vi "solar_write QTimerStopAll.vi"(8 "error in (no error)":errorcluster, 11 "solar in":refnum<class "solar.lvclass">) -> (0 "error out":errorcluster, 2 "Previously Running":bool[](array[boolean]), 3 "solar out":refnum<class "solar.lvclass">)   [LabVIEW 2018, in "solar.lvclass"]
doc: "This stops all QTimers registered and returns if the QTimer was prevously running prior to the stop."
uses:
  solar.lvclass
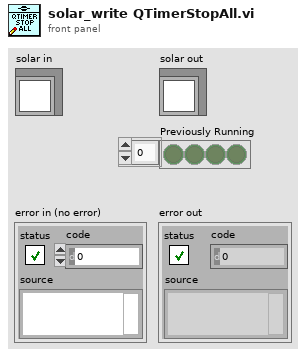
[diagram p1: front panel]
types:
  T1 = typedef "solar_ctl SOLAR Refnum.ctl" = refnum<k1>
  T2 = typedef "solar_ctl SOLAR Global.ctl" = cluster{"Targets":T3[], "AppDir":path, "solar.ini":path, "ConfigsDir":path, "CosmosDir":path, "LogsDir":path, "ExePath":path, "ExeVersion":string, "PartNum":string, "AppSetup":string, "Title":string, "Main.ini":path, "Temp.ini":path, "vSOLAR":string, "Splash.png":string, "SplashWait":i32, "SOLARUE":refnum<user-event>, "VoyagerRefnum":T4, "QTimerRefnum":T5}
  T3 = typedef "solar_ctl Target Global.ctl" = cluster{"Target":string, "Q":refnum<queue>, "UE":refnum<user-event>, "VI":refnum<vi>, "Menu":refnum<k9>, "Data":refnum<data-value>, "Attributes":variant}
  T4 = typedef "solar_voy_ctl Voyager Refnum.ctl" = refnum<k1>
  T5 = typedef "solar_qtimer_ctl Refnum.ctl" = refnum<k1>
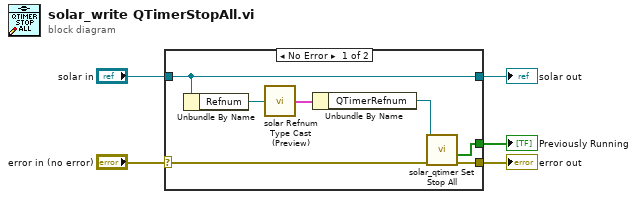
[diagram p0: block diagram]
diagram:
  n1 = case shown="No Error" "error in (no error)" {
    selector: "error in (no error)" -> [w9 w14]
    tunnel: "solar in" -> [w10 w13]
    tunnel: [w8 w14] -> w4
    tunnel: [w10 w13] -> w2
    tunnel: [w6 _] -> w1
    frame No Error {
      n2 = Unbundle By Name(w10) -> ("Refnum"=w12:T1)
      n3 = call "solar Refnum Type Cast (Preview).vi"("Refnum"=w12) -> ("SOLAR"=w11:T2)  [unwired: 8 in]
      n4 = Unbundle By Name(w11) -> ("QTimerRefnum"=w7:T5)
      n5 = call "solar_qtimer Set Stop All.vi"("error in (no error)"=w9, "QTimer Refnum in"=w7) -> ("error out"=w8:errorcluster, "Previously Running"=w6:bool[])  [unwired: 6 in, 2 out]
    }
    frame Error {
    }
  }
  "error out" <- w4
  "solar out" <- w2
  "Previously Running" <- w1
